vi "sensor_parameter_strings_to_strict_type.vi"(8 "error in (no error)":errorcluster, 10 "Sensor parameters (strings)":T2) -> (0 "error out":errorcluster, 2 "Sensor parameters":T1)   [LabVIEW 2018]
uses:
  sensor_parameters_strings.ctl
  sensor_parameters.ctl
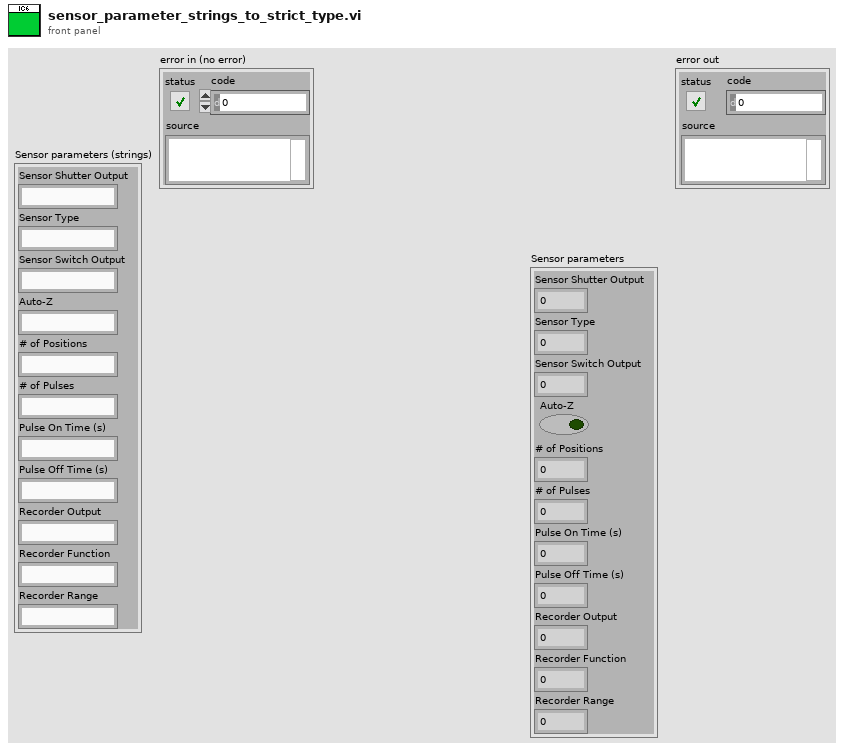
[diagram p1: front panel]
types:
  T1 = typedef "sensor_parameters.ctl" = cluster{"Sensor Shutter Output":u8, "Sensor Type":u8, "Sensor Switch Output":u8, "Auto-Z":bool, "# of Positions":u8, "# of Pulses":u8, "Pulse On Time (s)":sgl, "Pulse Off Time (s)":sgl, "Recorder Output":u8, "Recorder Function":u8, "Recorder Range":u32}
  T2 = typedef "sensor_parameters_strings.ctl" = cluster{"Sensor Shutter Output":string, "Sensor Type":string, "Sensor Switch Output":string, "Auto-Z":string, "# of Positions":string, "# of Pulses":string, "Pulse On Time (s)":string, "Pulse Off Time (s)":string, "Recorder Output":string, "Recorder Function":string, "Recorder Range":string}
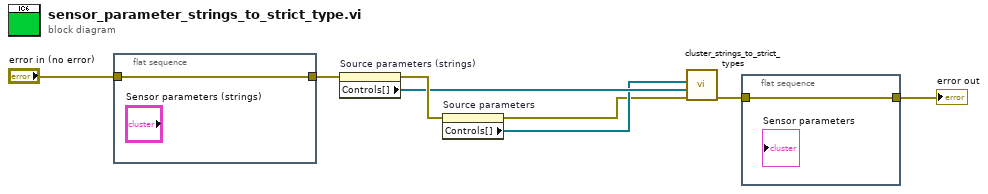
[diagram p0: block diagram]
diagram:
  n1 = flat-sequence {
    tunnel: "error in (no error)" -> [w9]
    tunnel: [w9] -> w6
    frame #0 {
    }
  }
  n2 = property on="Source parameters (strings)" class="Clust (strict)"(error in=w6) -> (error out=w5:errorcluster, "Controls[]"=w4:refnum<vi>[])  [unwired: 1 in, 1 out]
  n3 = property on="Source parameters" class="Clust (strict)"(error in=w5) -> (error out=w2:errorcluster, "Controls[]"=w3:refnum<vi>[])  [unwired: 1 in, 1 out]
  n4 = call "cluster_strings_to_strict_types.vi"("error in (no error)"=w2, "Controls[] (strings)"=w4, "Controls[]"=w3) -> ("error out"=w1:errorcluster)  [unwired: 8 in]
  n5 = flat-sequence {
    tunnel: w1 -> [w10]
    tunnel: [w10] -> w7
    frame #0 {
    }
  }
  "error out" <- w7
